vi "Untitled 2.vi"(8 "error in (no error)":errorcluster, 11 "Model in":refnum<class "Model.lvclass">) -> (0 "error out":errorcluster, 3 "Model out":refnum<class "Model.lvclass">)   [LabVIEW 2021, in "Model.lvlib" / "Model.lvclass"]
uses:
  Model.lvclass
  <userlib>/John_Lib/OPCUA/OPCUA.lvclass
  <userlib>/John_Lib/OPCUA/add NameSpace for single NoteID.vi
  <vilib>/OPCUA/client/internal/Read.vi
  <vilib>/OPCUA/client/internal/Read String.vi
  <vilib>/Utility/error.llb/Trim Whitespace.vi
  Model.lvclass/Model.ctl
panel:
  out "error out 3":errorcluster
  out "Numeric":i32
  out "value":string
  out "timestamp":timestamp
  in  "node ID":string
  in  "stop":bool
  out "error out 2":errorcluster
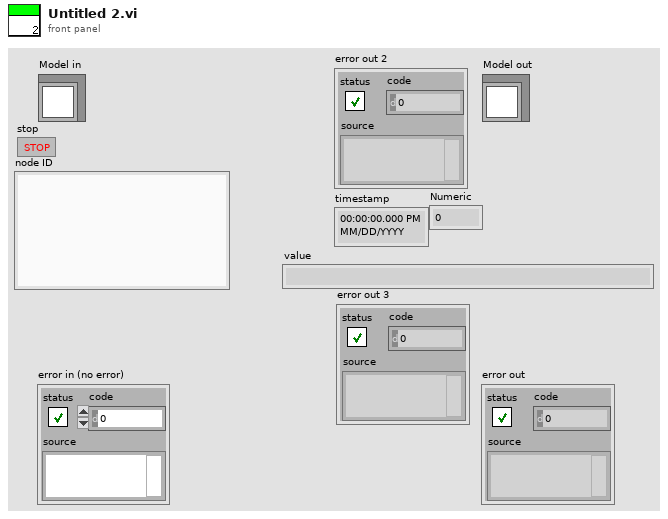
[diagram p1: front panel]
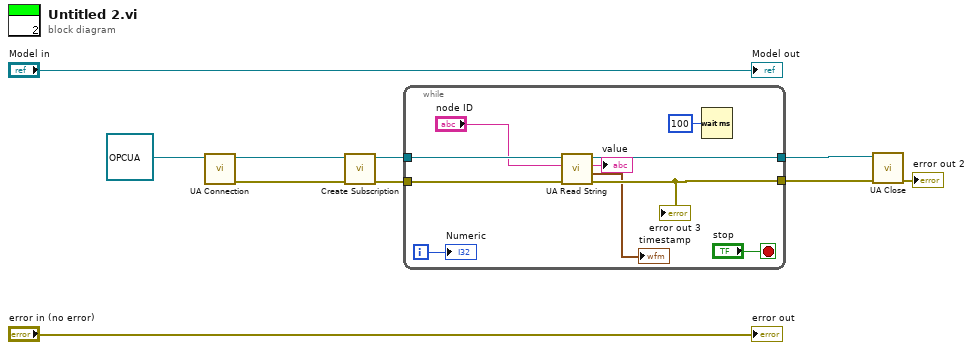
[diagram p0: block diagram]
diagram:
  n1 = call <userlib>:"UA Connection.vi"("OPCUA in"=refnum<class "OPCUA.lvclass"> refnum) -> ("error out"=w4:errorcluster, "OPCUA out"=w8:refnum<class "OPCUA.lvclass">)  [unwired: 9 in]
  n2 = call <userlib>:"Create Subscription.vi"("error in (no error)"=w4, "OPCUA in"=w8) -> ("error out"=w3:errorcluster, "OPCUA out"=w6:refnum<class "OPCUA.lvclass">)  [unwired: 7 in, 1 out]
  n3 = while {
    tunnel: w6 -> [w20]
    tunnel: [w19] -> w5
    tunnel: w3 -> [w18]
    tunnel: [w17] -> w2
    i -> [w11]
    stop <- "stop" stop-if-true
    n4 = call <userlib>:"UA Read String.vi"("error in (no error)"=w18, "node ID"="node ID", "OPCUA in"=w20) -> ("error out"=w17:errorcluster, "timestamp"=→"timestamp":timestamp, "value"=→"value":string, "OPCUA out"=w19:refnum<class "OPCUA.lvclass">)  [unwired: 4 in, 1 out]
    "error out 3" <- w17
    n5 = Wait (ms)(milliseconds to wait=u32 100) -> ()  [unwired: 1 out]
    "Numeric" <- w11
  }
  n6 = call <userlib>:"UA Close.vi"("error in (no error)"=w2, "OPCUA in"=w5) -> ("error out"=→"error out 2":errorcluster)  [unwired: 8 in, 1 out]
  "error out" <- "error in (no error)"
  "Model out" <- "Model in"
